vi "Get In Place Items Displayed.vi"(11 "Affected Items":T2) -> (3 "Displayed Items":T1[](array[typedef]))   [LabVIEW 2023]
doc: "Get input or outpur terminals displayed from a named bundler or unbundler. This is used for the dialog to remove and rearrange those items."
uses:
  top/BundleMagic.ctl
  Cluster Element Description.ctl
  <vilib>/Utility/Data Type/NI_Data Type.lvlib
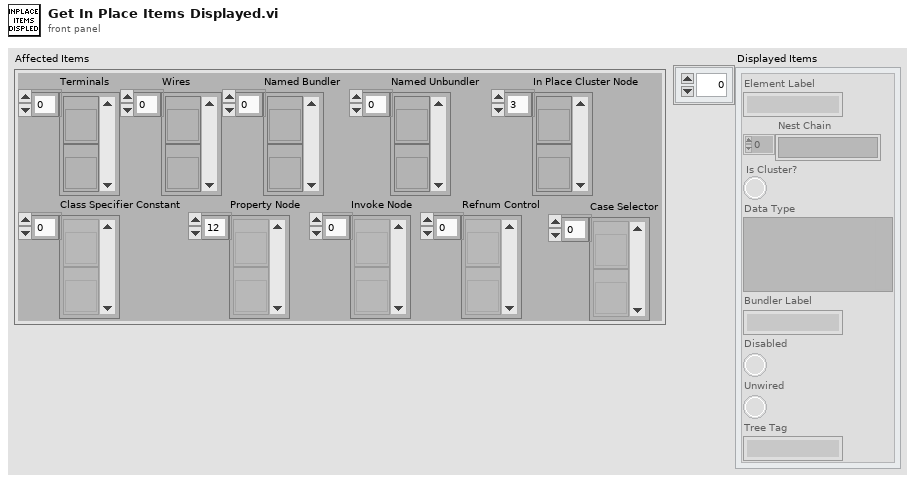
[diagram p1: front panel]
types:
  T1 = typedef "Cluster Element Description.ctl" = cluster{"Element Label":string, "Nest Chain":string[], "Is Cluster?":bool, "Data Type":variant, "Bundler Label":string, "Disabled":bool, "Unwired":bool, "Tree Tag":string}
  T2 = typedef "BundleMagic.ctl" = cluster{"Terminals":refnum<vi>[], "Wires":refnum<vi>[], "Named Bundler":refnum<vi>[], "Named Unbundler":refnum<vi>[], "In Place Cluster Node":refnum<vi>[], "Class Specifier Constant":refnum<vi>[], "Property Node":refnum<vi>[], "Invoke Node":refnum<vi>[], "Refnum Control":refnum<vi>[], "Case Selector":refnum<vi>[]}
  T3 = enum8{"Invalid Type", "Void", "I8", "I16", "I32", "I64", "U8", "U16", "U32", "U64", "Single Float", "Double Float", "Extended Float", "Single Complex", "Double Complex", "Extended Complex", "Enum U8", "Enum U16", "Enum U32", "Enum U64", "Single Float With Unit", "Double Float With Unit", "Extended Float With Unit", "Single Complex with Unit", "Double Complex with Unit", "Extended Complex with Unit", "Boolean", "String", "Path", "Picture", "Tag", "Array", "Cluster", "Variant", "LV Variant", "Waveform", "Timestamp", "Digital Waveform", "Digital Data", "ExpressData", "Refnum", "External Data", "VI", "Poly VI", "LabVIEW Class Instance", "Fixed Point"}
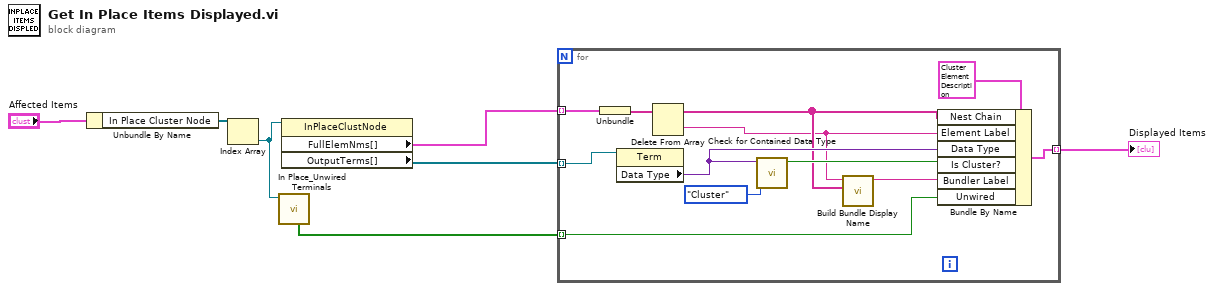
[diagram p0: block diagram]
diagram:
  n1 = Unbundle By Name("Affected Items") -> ("In Place Cluster Node"=w4:refnum<vi>[])
  n2 = Index Array(array=w4) -> (element=w2:refnum<vi>)  [unwired: 1 in]
  n3 = call "In Place_Unwired Terminals.vi"("In Place Node"=w2) -> ("Unwired?"=w1:bool[])  [unwired: 6 in, 4 out]
  n4 = property class="InPlaceClustNode"(reference=w2) -> ("FullElemNms[]"=w3:cluster{string[]}[], "OutputTerms[]"=w7:refnum<vi>[])  [unwired: 1 in, 2 out]
  n5 = for {
    tunnel: w7 -> [w19] mode=indexing
    tunnel: [w17] -> w6 mode=indexing
    tunnel: w3 -> [w16] mode=indexing
    tunnel: w1 -> [w8] mode=indexing
    n6 = Unbundle(w16) -> (w15:string[])
    n7 = property class="Term"(reference=w19) -> ("Data Type"=w14:variant)  [unwired: 1 in, 2 out]
    n8 = Delete From Array(array=w15) -> (deleted portion=w10:string, array with subset deleted=w11:string[])  [unwired: 2 in]
    n9 = call <vilib>:"Check for Contained Data Type.vi"("data type to find"=T3."Cluster", "variant"=w14) -> ("contains data type to find?"=w12:bool)  [unwired: 8 in, 1 out]
    n10 = call "Build Bundle Display Name.vi"("Nest Chain"=w11, "Element Label"=w10) -> ("Bundle display name"=w9:string)  [unwired: 9 in]
    n11 = Bundle By Name(cluster=T1 {"Element Label"="", "Nest Chain"=[], "Is Cluster?"=FALSE, "Data Type"=variant, "Bundler Label"="", "Disabled"=FALSE, "Unwired"=FALSE, "Tree Tag"=""} ("Cluster"), "Nest Chain"=w11, "Element Label"=w10, "Data Type"=w14, "Is Cluster?"=w12, "Bundler Label"=w9, "Unwired"=w8) -> (w17:T1)
  }
  "Displayed Items" <- w6
